vi "Global Distance.vi"() -> ()   [LabVIEW 2015]
panel:
  in  "LLS":dbl
  in  "RLS":dbl
  in  "delta3":dbl
  in  "dz":dbl
  in  "delta2":dbl
  in  "delta1":dbl
  in  "dy":dbl
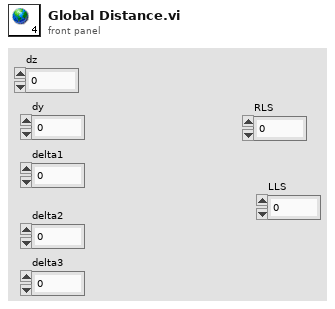
[diagram p1: front panel]
diagram:
